vi "Cal.vi"(8 "error in (no error)":errorcluster, 9 "b":dbl, 10 "a":dbl, 11 "Add in":refnum<class "Add.lvclass">) -> (0 "error out":errorcluster, 2 "Result":dbl, 3 "Add out":refnum<class "Add.lvclass">)   [LabVIEW 2014, in "Caculator.lvlib" / "Add.lvclass"]
uses:
  Add.lvclass
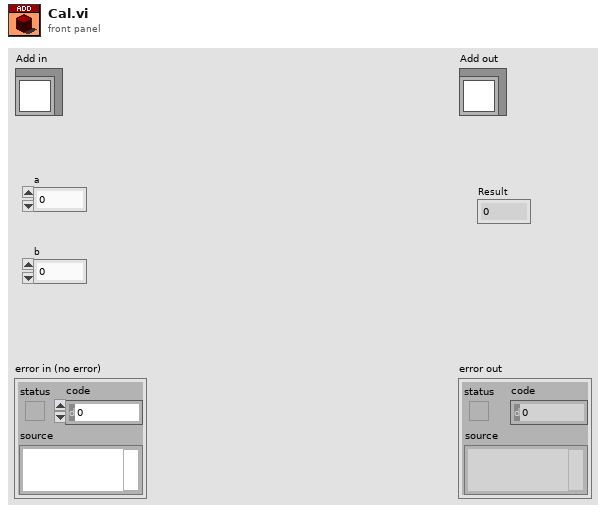
[diagram p1: front panel]
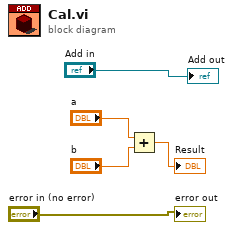
[diagram p0: block diagram]
diagram:
  n1 = Add(x="a", y="b") -> (x+y=→"Result":dbl)
  "error out" <- "error in (no error)"
  "Add out" <- "Add in"
